vi "Convert Timestamped Packets.vi"(0 "timestamped llp packet":T2={"timestamp"={"valid"=FALSE, "count"=0.0, "id"=enum."SI0 LLP", "metadata"=0}, "llp packet"={"header"={"word count"=0, "ecc"=0.0, "vcx"=0.0, "data type"=0.0, "vc"=0.0}, "header valid"=FALSE, "payload"={"end of payload"=FALSE, "end of payload index"=0.0, "payload data"=[0, 0, 0, 0]}, "payload valid"=FALSE, "footer"={"crc"=0}, "footer valid"=FALSE, "end of packet"=FALSE}}, 1 "reset":bool, 9 "input valid":bool, 12 "ready for ouput":bool) -> (4 "tagged llp packet":T9={"tag"={"timestamp"={"valid"=FALSE, "count"=0.0, "id"=enum."SI0 LLP", "metadata"=0}, "size"={"bytes"=0.0, "valid"=FALSE}}, "llp packet"={"header"={"word count"=0, "ecc"=0.0, "vcx"=0.0, "data type"=0.0, "vc"=0.0}, "header valid"=FALSE, "payload"={"end of payload"=FALSE, "end of payload index"=0.0, "payload data"=[0, 0, 0, 0]}, "payload valid"=FALSE, "footer"={"crc"=0}, "footer valid"=FALSE, "end of packet"=FALSE}}, 8 "dram status":T1, 10 "output valid":bool, 14 "ready for input":bool)   [LabVIEW 2020, in "GettingStarted_Acq_Tap_148X_FPGA.lvlib"]
uses:
  GettingStarted_Acq_Tap_148X_FPGA.lvlib
  <instrlib>/FlexRIO/CSI-2/v2/FPGA/Types/Tagged LLP Packet.ctl
  <instrlib>/FlexRIO/CSI-2/v2/FPGA/Types/FPGA LLP Packet Tag.ctl
  <instrlib>/FlexRIO/CSI-2/v2/FPGA/Types/FPGA LLP Packet Timestamp.ctl
  <instrlib>/FlexRIO/CSI-2/v2/FPGA/Types/Timestamp ID.ctl
  <instrlib>/FlexRIO/CSI-2/v2/FPGA/Types/FPGA LLP Packet Size.ctl
  <instrlib>/FlexRIO/CSI-2/v2/FPGA/Types/LLP Packet.ctl
  <instrlib>/FlexRIO/CSI-2/v2/FPGA/Types/LLP Packet Header.ctl
  <instrlib>/FlexRIO/CSI-2/v2/FPGA/Types/LLP Packet Payload.ctl
  <instrlib>/FlexRIO/CSI-2/v2/FPGA/Types/LLP Packet Footer.ctl
  <instrlib>/FlexRIO/CSI-2/v2/FPGA/Types/Timestamped LLP Packet.ctl
  Common/Types/DRAM Status.ctl
  <instrlib>/FlexRIO/CSI-2/v2/FPGA/NI CSI-2 API FPGA v2.lvlib
  Common/GettingStarted_Common_148X_FPGA.lvlib
panel:
  out "in reset":bool
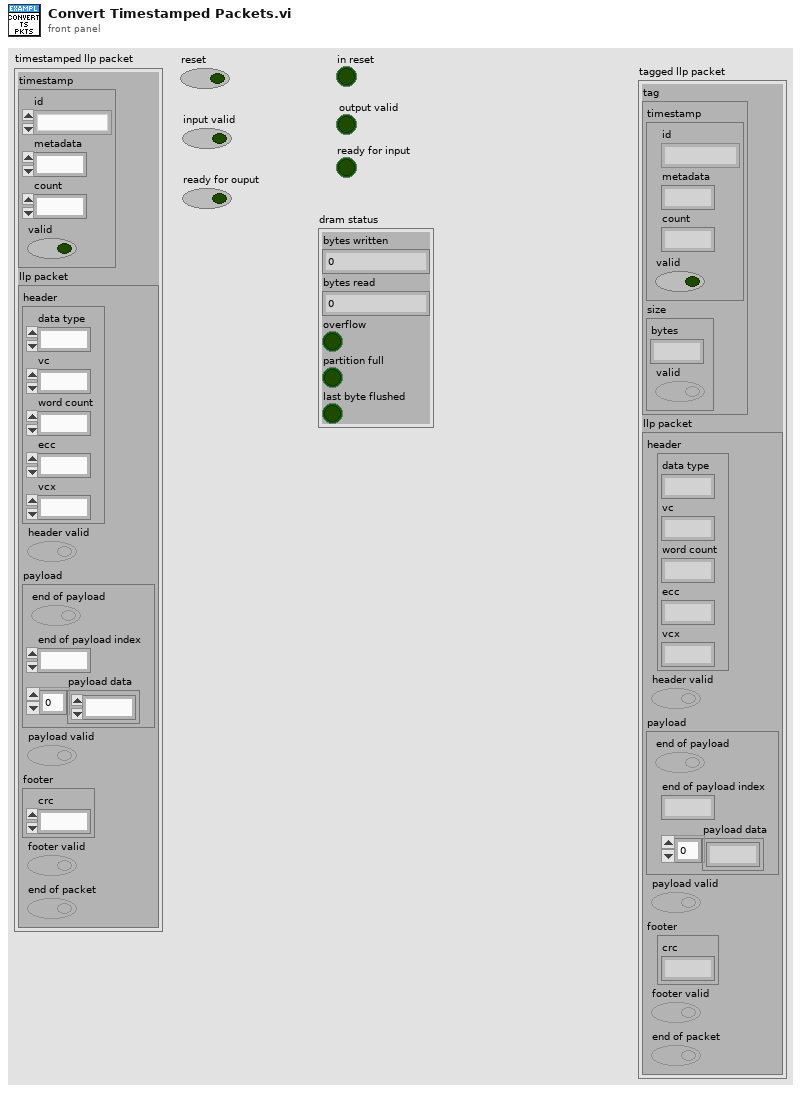
[diagram p1: front panel]
types:
  T1 = typedef "GettingStarted_Common_148X_FPGA.lvlib/DRAM Status.ctl" = cluster{"bytes written":u64, "bytes read":u64, "overflow":bool, "partition full":bool, "last byte flushed":bool}
  T2 = typedef "NI CSI-2 API FPGA v2.lvlib/Timestamped LLP Packet.ctl" = cluster{"timestamp":T3, "llp packet":T5}
  T3 = typedef "NI CSI-2 API FPGA v2.lvlib/FPGA LLP Packet Timestamp.ctl" = cluster{"valid":bool, "count":fxp<+,50,50>, "id":T4, "metadata":u8}
  T4 = typedef "NI CSI-2 API FPGA v2.lvlib/Timestamp ID.ctl" = enum8{"SI0 LLP", "SI1 LLP", "SI2 LLP", "SI3 LLP", "SI4 LLP", "SI5 LLP", "SI6 LLP", "SI7 LLP", "SO0 LLP", "SO1 LLP", "SO2 LLP", "SO3 LLP", "SO4 LLP", "SO5 LLP", "SO6 LLP", "SO7 LLP", "Ser0 GPIO Bank", "Ser1 GPIO Bank", "Ser2 GPIO Bank", "Ser3 GPIO Bank", "Ser4 GPIO Bank", "Ser5 GPIO Bank", "Ser6 GPIO Bank", "Ser7 GPIO Bank", "Des0 GPIO Bank", "Des1 GPIO Bank", "Des2 GPIO Bank", "Des3 GPIO Bank", "Des4 GPIO Bank", "Des5 GPIO Bank", "Des6 GPIO Bank", "Des7 GPIO Bank", "User0", "User1", "User2", "User3", "User4", "User5", "User6", "User7", "User8", "User9", "User10", "User11", "User12", "User13", "User14", "User15", "User16", "User17", "User18", "User19", "User20", "User21", "User22", "User23", "User24", "User25", "User26", "User27", "User28", "User29", "User30", "User31"}
  T5 = typedef "NI CSI-2 API FPGA v2.lvlib/LLP Packet.ctl" = cluster{"header":T6, "header valid":bool, "payload":T7, "payload valid":bool, "footer":T8, "footer valid":bool, "end of packet":bool}
  T6 = typedef "NI CSI-2 API FPGA v2.lvlib/LLP Packet Header.ctl" = cluster{"word count":u16, "ecc":fxp<+,6,6>, "vcx":fxp<+,2,2>, "data type":fxp<+,6,6>, "vc":fxp<+,2,2>}
  T7 = typedef "NI CSI-2 API FPGA v2.lvlib/LLP Packet Payload.ctl" = cluster{"end of payload":bool, "end of payload index":fxp<+,3,3>, "payload data":u8[]}
  T8 = typedef "NI CSI-2 API FPGA v2.lvlib/LLP Packet Footer.ctl" = cluster{"crc":u16}
  T9 = typedef "NI CSI-2 API FPGA v2.lvlib/Tagged LLP Packet.ctl" = cluster{"tag":T10, "llp packet":T5}
  T10 = typedef "NI CSI-2 API FPGA v2.lvlib/FPGA LLP Packet Tag.ctl" = cluster{"timestamp":T3, "size":T11}
  T11 = typedef "NI CSI-2 API FPGA v2.lvlib/FPGA LLP Packet Size.ctl" = cluster{"bytes":fxp<+,17,17>, "valid":bool}
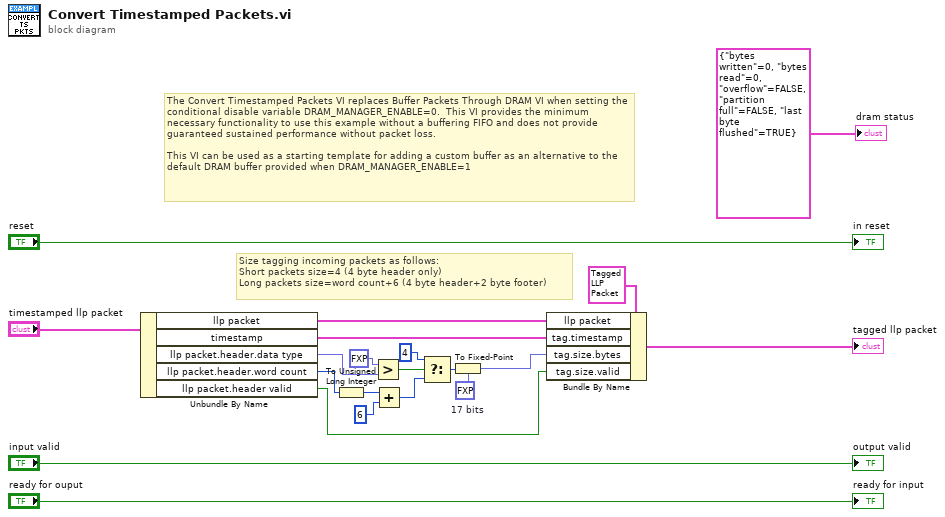
[diagram p0: block diagram]
diagram:
  w9 = fxp<+,17,17> 0.0  # 17 bits
  # "Size tagging incoming packets as follows:\nShort packets size=4 (4 byte header only)\nLong packets size=word count+6 (4 byte header+2 byte footer)"
  # "The Convert Timestamped Packets VI replaces Buffer Packets Through DRAM VI when setting the conditional disable variable DRAM_MANAGER_ENABLE=0.  This VI provides the minimum necessary functionality to use this example without a buffering FIFO and does not provide guaranteed sustained performance without packet loss.\n\nThis VI can be used as a starting template for adding a custom buffer as an alternative to the default DRAM buffer provided when DRAM_MANAGER_ENABLE=1"
  n1 = Unbundle By Name("timestamped llp packet") -> ("llp packet"=w20:T5, "timestamp"=w19:T3, "llp packet.header.data type"=w17:fxp<+,6,6>, "llp packet.header.word count"=w14:u16, "llp packet.header valid"=w6:bool)
  n2 = To Unsigned Long Integer(number=w14) -> (unsigned 32bit integer=w13:u32)
  n3 = Greater?(x=fxp<+,6,6> 16.0 ("y"), y=w17) -> (0:w15:bool)
  n4 = Add(x=w13, y=u32 6 ("llp packet.header.word count")) -> (x+y=w11:u32)
  n5 = Select(t=u32 4, s=w15, f=w11) -> (s? t:f=w8:u32)
  n6 = To Fixed-Point(fixed-point type=w9, number=w8) -> (fixed-point=w7:fxp<+,17,17>)
  n7 = Bundle By Name(cluster=T9 {"tag"={"timestamp"={"valid"=FALSE, "count"=0.0, "id"=enum."SI0 LLP", "metadata"=0}, "size"={"bytes"=0.0, "valid"=FALSE}}, "llp packet"={"header"={"word count"=0, "ecc"=0.0, "vcx"=0.0, "data type"=0.0, "vc"=0.0}, "header valid"=FALSE, "payload"={"end of payload"=FALSE, "end of payload index"=0.0, "payload data"=[]}, "payload valid"=FALSE, "footer"={"crc"=0}, "footer valid"=FALSE, "end of packet"=FALSE}} ("tagged llp packet"), "llp packet"=w20, "tag.timestamp"=w19, "tag.size.bytes"=w7, "tag.size.valid"=w6) -> (→"tagged llp packet":T9)
  "ready for input" <- "ready for ouput"
  "in reset" <- "reset"
  "output valid" <- "input valid"
  "dram status" <- T1 {"bytes written"=0, "bytes read"=0, "overflow"=FALSE, "partition full"=FALSE, "last byte flushed"=TRUE} ("dram status")
